vi "Get Settings.vi"(0 "Font Settings in":refnum<class "Font Settings.lvclass">) -> (1 "Font Path":path, 2 "Font Name":string, 3 "Size":dbl)   [LabVIEW 2023, in "Glyph Drawer.lvlib" / "Font Settings.lvclass"]
uses:
  Font Settings.lvclass
  Font Settings.lvclass/Font Settings.ctl
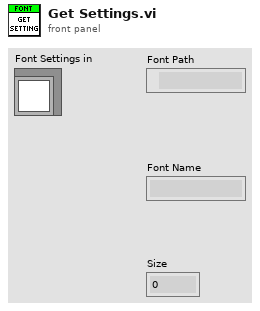
[diagram p1: front panel]
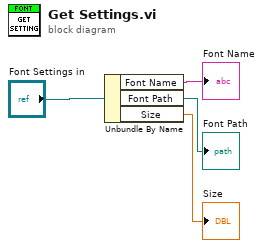
[diagram p0: block diagram]
diagram:
  n1 = Unbundle By Name("Font Settings in") -> ("Font Name"=→"Font Name":string, "Font Path"=→"Font Path":path, "Size"=→"Size":dbl)
